vi "Stop after trigger.vi"(6 "reset":bool, 9 "delay after trigger":i64, 10 "current time":i64, 11 "trigger":bool) -> (3 "done":bool)   [LabVIEW 2013]
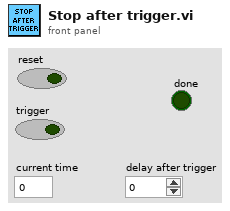
[diagram p1: front panel]
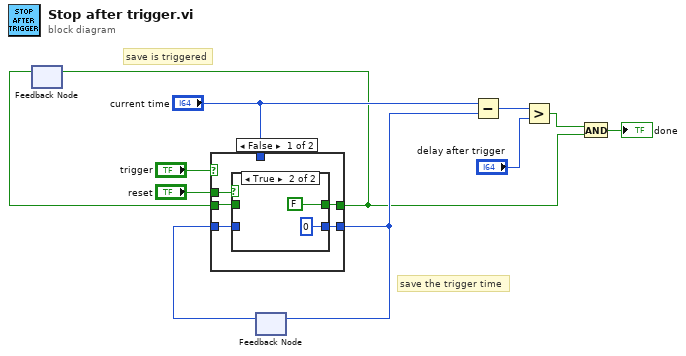
[diagram p0: block diagram]
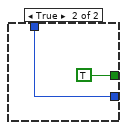
[diagram p3: hidden frame]
diagram:
  # "save the trigger time"
  # "save is triggered"
  n1 = feedback #1() -> (w4:bool)  [unwired: 1 in]
  n2 = feedback #2() -> (w10:u64)  [unwired: 1 in]
  n3 = case shown="False" "trigger" {
    tunnel: [w15 TRUE] -> w1
    tunnel: "current time" -> [_ w21]
    tunnel: [w12 w21] -> w8
    tunnel: w10 -> [w13 _]
    tunnel: "reset" -> [w16 _]
    tunnel: w4 -> [w14 _]
    frame False {
      n4 = case shown="True" w16 {
        tunnel: [w18 FALSE] -> w15
        tunnel: w14 -> [w18 _]
        tunnel: w13 -> [w17 _]
        tunnel: [w17 u64 0 ("time")] -> w12
        frame False {
        }
        frame True {
        }
      }
    }
    frame True {
    }
  }
  n5 = feedback-in #1(w1) -> ()
  n6 = feedback-in #2(w8) -> ()
  n7 = Subtract(x="current time", y=w8) -> (x-y=w7:u64)
  n8 = Greater?(x=w7, y="delay after trigger") -> (0:w2:bool)
  n9 = And(x=w2, y=w1) -> (x .and. y?=→"done":bool)
